vi "FG - DbgTimers Class Ref.vi"(0 "DbgTimers in":refnum<class "DbgTimers.lvclass">, 1 "error in (no error)":errorcluster, 4 "action (Get)":T1=enum."Get") -> (7 "DbgTimers out":refnum<class "DbgTimers.lvclass">, 8 "error out":errorcluster)   [LabVIEW 2017, in "DbgTimers.lvclass"]
doc: "Developed by Kevin Thompson\nkevin@thompsonengineering.net\n\nCopyright 2018-2020\nThompson Engineering, LLC"
uses:
  DbgTimers.lvclass
  Ichor_Common/DataTypes/TD GetSet ActionSelect--enum.ctl
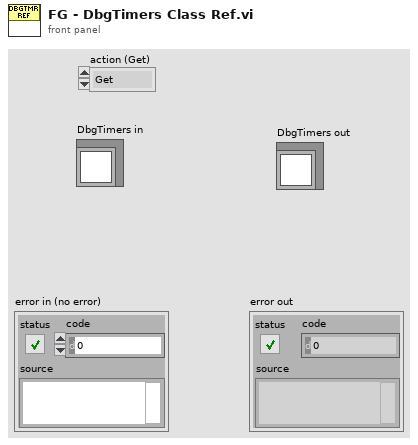
[diagram p1: front panel]
types:
  T1 = typedef "TD GetSet ActionSelect--enum.ctl" = enum16{"Init", "Get", "Set"}
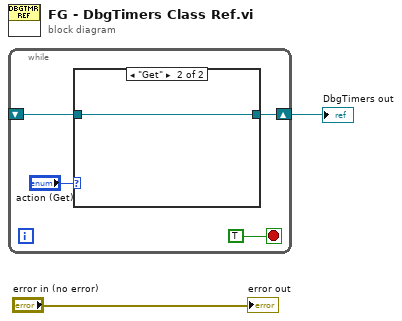
[diagram p0: block diagram]
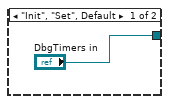
[diagram p2: hidden frame]
diagram:
  n1 = while {
    shift-right: [w4] -> w2
    shift-left: _ -> [w3]
    stop <- TRUE stop-if-true
    n2 = case shown="\"Get\"" "action (Get)" {
      tunnel: ["DbgTimers in" w8] -> w4
      tunnel: w3 -> [_ w8]
      frame "Init", "Set", Default {
      }
      frame "Get" {
      }
    }
  }
  "DbgTimers out" <- w2
  "error out" <- "error in (no error)"
